vi "Step enumeration.vi"(11 "SweepProperties":T1) -> (3 "Step N of 131,072":i32)   [LabVIEW 2018]
doc: "Phase Shift and Attenuation values are hardcoded here.\nindexing will not work if test builder list boxes are changed."
uses:
  SearchableTag.ctl
  Sequence/SequenceSubvis/RF Direction.ctl
  Sequence/SequenceSubvis/PolarizationSelect.ctl
  DataLog.lvclass
panel:
  out "step within 4096 scale":i32
  out "size(s)":i32
  out "index of Atten":i32
  out "index of PS":i32
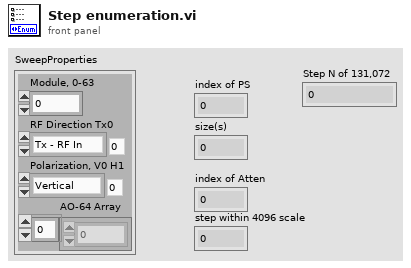
[diagram p1: front panel]
types:
  T1 = typedef "DataLog.lvclass/SearchableTag.ctl" = cluster{"Module, 0-63":i32, "RF Direction Tx0":T2, "Polarization, V0 H1":T3, "AO-64 Array":dbl[]}
  T2 = typedef "RF Direction.ctl" = enum16{"Tx - RF In", "Rx - RF Out"}
  T3 = typedef "PolarizationSelect.ctl" = enum16{"Vertical", "Horizontal"}
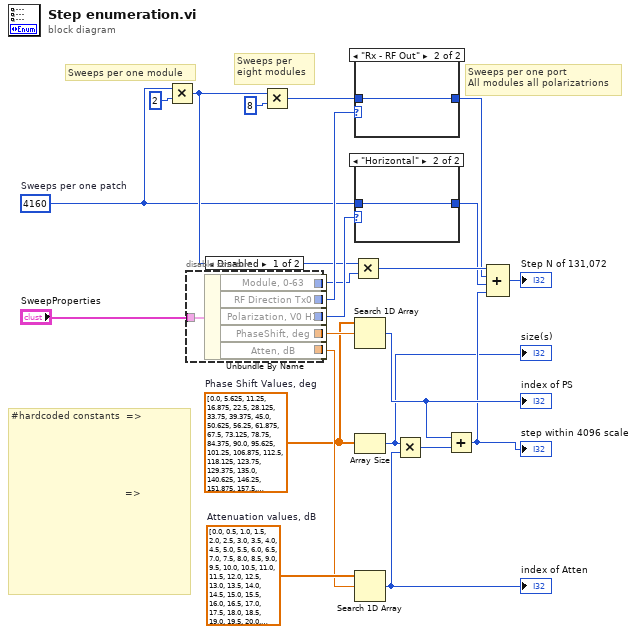
[diagram p0: block diagram]
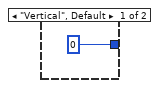
[diagram p3: hidden frame]
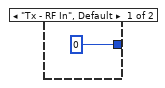
[diagram p4: hidden frame]
diagram:
  w1 = 4160  # Sweeps per one patch
  w17 = dbl[] [0.0, 0.5, 1.0, 1.5, 2.0, 2.5, 3.0, 3.5, 4.0, 4.5, 5.0, 5.5, 6.0, 6.5, 7.0, 7.5, 8.0, 8.5, 9.0, 9.5, 10.0, 10.5, 11.0, 11.5, 12.0, 12.5, 13.0, 13.5, 14.0, 14.5, 15.0, 15.5, 16.0, 16.5, 17.0, 17.5, 18.0, 18.5, 19.0, 19.5, 20.0, 20.5, 21.0, 21.5, 22.0, 22.5, 23.0, 23.5, 24.0, 24.5, 25.0, 25.5, 26.0, 26.5, 27.0, 27.5, 28.0, 28.5, 29.0, 29.5, 30.0, 30.5, 31.0, 31.5]  # Attenuation values, dB
  w15 = dbl[] [0.0, 5.625, 11.25, 16.875, 22.5, 28.125, 33.75, 39.375, 45.0, 50.625, 56.25, 61.875, 67.5, 73.125, 78.75, 84.375, 90.0, 95.625, 101.25, 106.875, 112.5, 118.125, 123.75, 129.375, 135.0, 140.625, 146.25, 151.875, 157.5, 163.125, 168.75, 174.375, 180.0, 185.625, 191.25, 196.875, 202.5, 208.125, 213.75, 219.375, 225.0, 230.625, 236.25, 241.875, 247.5, 253.125, 258.75, 264.375, 270.0, 275.625, 281.25, 286.875, 292.5, 298.125, 303.75, 309.375, 315.0, 320.625, 326.25, 331.875, 337.5, 343.125, 348.75, 354.375, 359.0]  # Phase Shift Values, deg
  # "#hardcoded constants  =>\n\n\n\n\n\n\n                                      =>"
  # "Sweeps per \neight modules"
  # "Sweeps per one port\nAll modules all polarizatrions"
  # "Sweeps per one module"
  n1 = Multiply(x=w1, y=2) -> (x*y=w4:i32)
  n2 = disable-structure shown="Disabled" {
    disable-tunnel: "SweepProperties" -> [w28 _]
    disable-tunnel: [w27 _] -> w21
    disable-tunnel: [w26 _] -> w20
    disable-tunnel: [w25 _] -> w19
    disable-tunnel: [w24 _] -> w18
    disable-tunnel: [w23 _] -> w16
    frame Disabled {
      n3 = Unbundle By Name(w28) -> ("Module, 0-63"=w25:i32, "RF Direction Tx0"=w27:T2, "Polarization, V0 H1"=w26:T3, "PhaseShift, deg"=w24:dbl, "Atten, dB"=w23:dbl)
    }
    frame Enabled {
    }
  }
  n4 = Multiply(x=w4, y=8) -> (x*y=w2:i32)
  n5 = Multiply(x=w4, y=w19) -> (x*y=w11:i32)
  n6 = case shown="\"Rx - RF Out\"" w21 {
    tunnel: [0 w30] -> w10
    tunnel: w2 -> [_ w30]
    frame "Tx - RF In", Default {
    }
    frame "Rx - RF Out" {
    }
  }
  n7 = case shown="\"Horizontal\"" w20 {
    tunnel: [0 w32] -> w9
    tunnel: w1 -> [_ w32]
    frame "Vertical", Default {
    }
    frame "Horizontal" {
    }
  }
  n8 = Search 1D Array(1D array=w15, element=w18) -> (index of element=w13:i32)  [unwired: 1 in]
  "index of PS" <- w13
  n9 = Array Size(array=w15) -> (size(s)=w6:i32)
  "size(s)" <- w6
  n10 = Search 1D Array(1D array=w17, element=w16) -> (index of element=w12:i32)  [unwired: 1 in]
  "index of Atten" <- w12
  n11 = Multiply(x=w6, y=w12) -> (x*y=w14:i32)
  n12 = Add(x=w13, y=w14) -> (x+y=w8:i32)
  "step within 4096 scale" <- w8
  n13 = Compound Arithmetic op=ADD(w11, w10, w9, w8) -> (→"Step N of 131,072":i32)
